vi "全局变量.vi"() -> ()   [LabVIEW 2016, in "数据查询.lvlib"]
panel:
  in  "访问共享数据":bool
  out "配置文件 path":path
  out "create table":bool
  in  "ping":bool
  in  "选择界面":T1=enum."仪器数据"
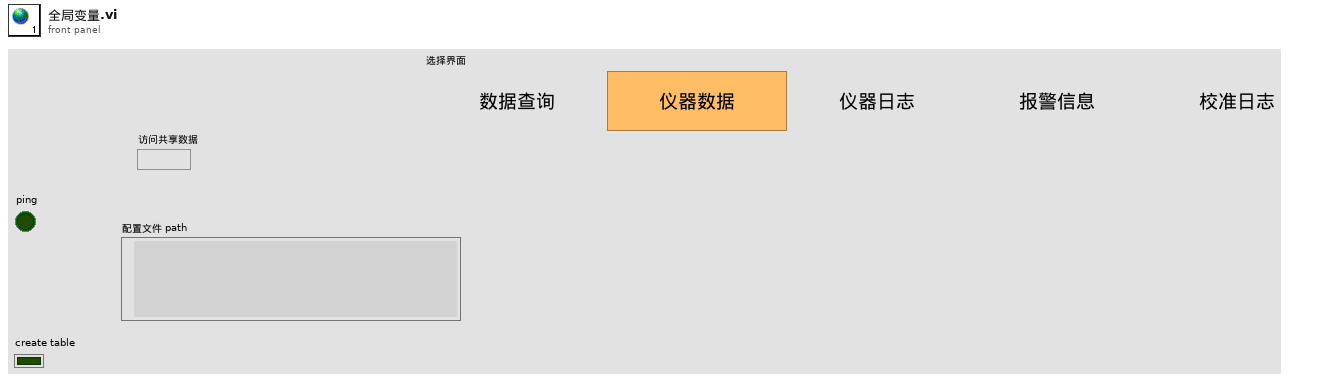
[diagram p1: front panel]
types:
  T1 = typedef "数据查询.lvlib/数据查询单选控件.ctl" = enum32{"数据查询", "仪器数据", "仪器日志", "报警信息", "校准日志"}
diagram:
